vi "AVI-Compatibility mode handler.vi"(10 "Initialisation message":bool) -> (1 "Cancelled":bool)   [LabVIEW 2013]
uses:
  Typedefs/AVI implementation enum.ctl
panel:
  out "AVI mode (out)":T1=enum."AVI2"
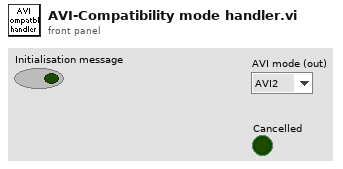
[diagram p1: front panel]
types:
  T1 = typedef "AVI implementation enum.ctl" = enum16{"AVI1", "AVI2"}
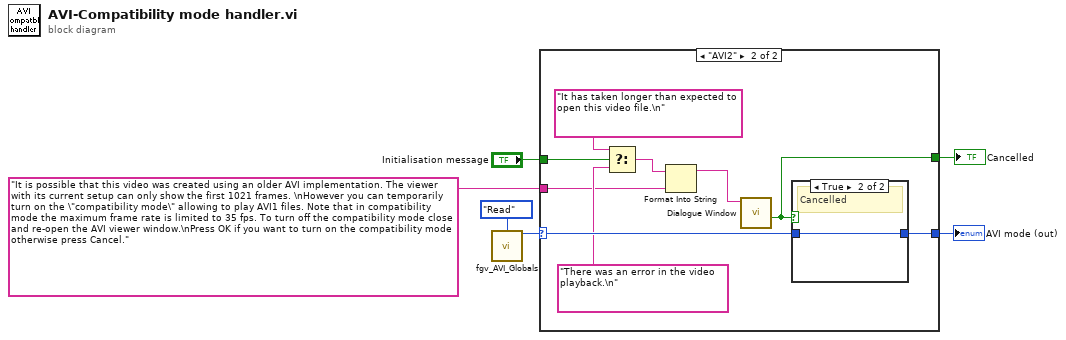
[diagram p0: block diagram]
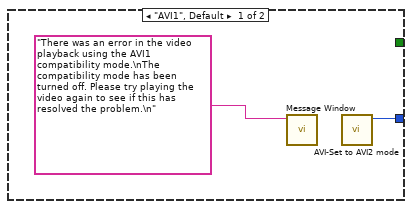
[diagram p2: hidden frame]
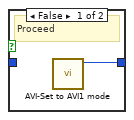
[diagram p3: hidden frame]
diagram:
  n1 = call "fgv_AVI_Globals.vi"("Function"=enum16{"Intialize", "Write", "Read", "Clear"}."Read") -> ("AVI mode"=w6:T1)  [unwired: 11 in, 3 out]
  n2 = case shown="\"AVI2\"" w6 {
    selector: w6 -> [_ w16]
    tunnel: [w7 w17] -> w4
    tunnel: "Initialisation message" -> [_ w15]
    tunnel: [_ w14] -> w2
    tunnel: "It is possible that this video was created using an older AVI implementation. The viewer with its current setup can only show the first 1021 frames. \nHowever you can temporarily turn on the \"compatibility mode\" allowing to play AVI1 files. Note that in compatibility mode the maximum frame rate is limited to 35 fps. To turn off the compatibility mode close and re-open the AVI viewer window.\nPress OK if you want to turn on the compatibility mode otherwise press Cancel." ("Message string") -> [_ w11]
    frame "AVI1", Default {
      n3 = call "Message Window.vi"("Message string"="There was an error in the video playback using the AVI1 compatibility mode.\nThe compatibility mode has been turned off. Please try playing the video again to see if this has resolved the problem.\n") -> ()  [unwired: 10 in, 1 out]
      n4 = call "AVI-Set to AVI2 mode.vi"() -> ("AVI mode"=w7:T1)  [unwired: 11 in]
    }
    frame "AVI2" {
      n5 = Select(t="It has taken longer than expected to open this video file.\n" ("Message string"), s=w15, f="There was an error in the video playback.\n" ("Message string")) -> (s? t:f=w10:string)
      n6 = Format Into String(initial string=w10, w11) -> (resulting string=w9:string)  [unwired: 2 in, 1 out]
      n7 = call "Dialogue Window.vi"("Message string"=w9) -> ("Cancelled (Left button pressed)"=w14:bool)  [unwired: 8 in, 2 out]
      n8 = case shown="True" w14 {
        tunnel: [w18 w19] -> w17
        tunnel: w16 -> [_ w19]
        frame False {
          # "Proceed"
          n9 = call "AVI-Set to AVI1 mode.vi"() -> ("AVI mode"=w18:T1)  [unwired: 11 in]
        }
        frame True {
          # "Cancelled"
        }
      }
    }
  }
  "AVI mode (out)" <- w4
  "Cancelled" <- w2
